vi "Test SLL DVR API Generator.vi"(6 "DVR API Suffix":string=" API", 8 "error in (no error)":errorcluster, 9 "DVR API Folder Name":string="DVR", 10 "Method Folder Name":string="Methods", 11 "Class Path":path=path "My Sample Class.lvclass") -> (0 "error out":errorcluster)   [LabVIEW 2016, in "SLL Scripting.lvlib"]
uses:
  SLL Scripting.lvlib
  SLL Class DVR API Generator.lvlib
  SLL File IO/SLL File IO.lvlib
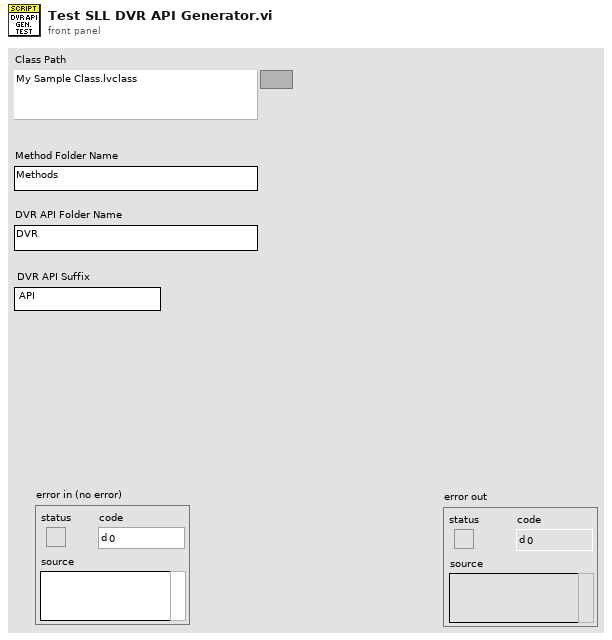
[diagram p1: front panel]
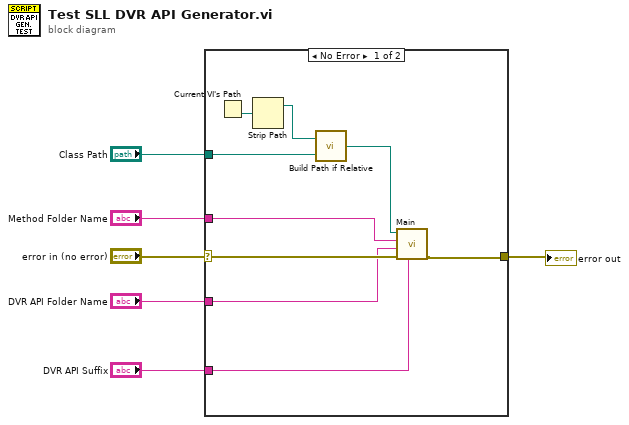
[diagram p0: block diagram]
diagram:
  n1 = case shown="No Error" "error in (no error)" {
    selector: "error in (no error)" -> [w15 w16]
    tunnel: [w14 w16] -> w5
    tunnel: "Class Path" -> [w11 _]
    tunnel: "DVR API Suffix" -> [w13 _]
    tunnel: "Method Folder Name" -> [w8 _]
    tunnel: "DVR API Folder Name" -> [w7 _]
    frame No Error {
      n2 = Current VI's Path() -> (path=w12:path)
      n3 = Strip Path(path=w12) -> (stripped path=w9:path)  [unwired: 1 out]
      n4 = call "Build Path if Relative.vi"("Relative or Absolute Path"=w11, "Base Path"=w9) -> ("Path Out"=w10:path)
      n5 = call "Main.vi"("DVR API Suffix"=w13, "error in (no error)"=w15, "DVR API Folder Name"=w7, "Method Folder Name"=w8, "Class Path"=w10) -> ("error out"=w14:errorcluster)  [unwired: 6 in]
    }
    frame Error {
    }
  }
  "error out" <- w5
